vi "HW2.3.vi"() -> ()   [LabVIEW 2014]
panel:
  out "sorted":cluster{"garde":dbl, i32}[](array[cluster])
  out "Numeric":dbl
  out "Numeric 2":dbl
  out "orignal":cluster{"grade":dbl, "ID number":i32}[](array[cluster])
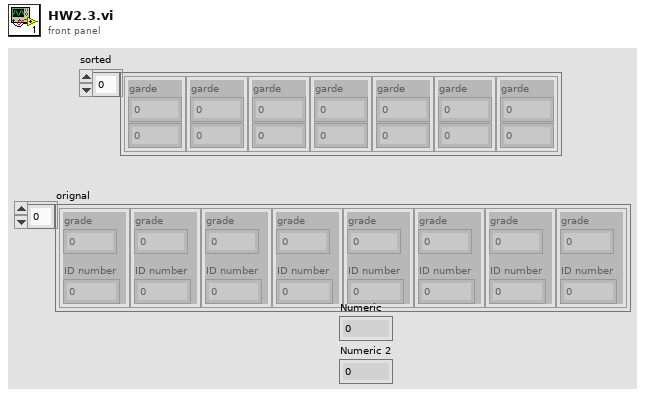
[diagram p1: front panel]
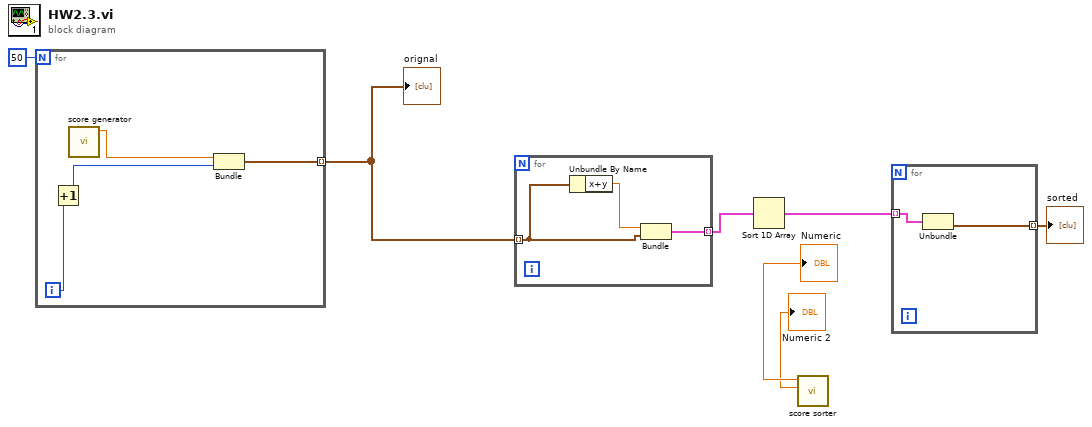
[diagram p0: block diagram]
diagram:
  n1 = for {
    N: 50 -> [_]
    tunnel: [w8] -> w6 mode=indexing
    i -> [w10]
    n2 = Increment(x=w10) -> (x+1=w9:i32)
    n3 = call "score generator.vi"() -> ("x+y"=w11:dbl)  [unwired: 11 in]
    n4 = Bundle("x+y"=w11, w9) -> (w8:cluster{"x+y":dbl, i32})  [unwired: 1 in]
  }
  "orignal" <- w6
  n5 = for {
    tunnel: w6 -> [w13] mode=indexing
    tunnel: [w12] -> w3 mode=indexing
    n6 = Unbundle By Name(w13) -> ("x+y"=w14:dbl)
    n7 = Bundle("x+y"=w14, w13) -> (w12:cluster{"x+y":dbl, cluster{"x+y":dbl, i32}})  [unwired: 1 in]
  }
  n8 = Sort 1D Array(array=w3) -> (sorted array=w2:cluster{"x+y":dbl, cluster{"x+y":dbl, i32}}[])
  n9 = call "score sorter.vi"() -> ("Numeric 2"=→"Numeric 2":dbl, "Numeric"=→"Numeric":dbl)  [unwired: 9 in, 1 out]
  n10 = for {
    tunnel: w2 -> [w16] mode=indexing
    tunnel: [w15] -> w1 mode=indexing
    n11 = Unbundle(w16) -> (w15:cluster{"x+y":dbl, i32})  [unwired: 1 out]
  }
  "sorted" <- w1
